vi "XNET.Cluster.Convert.Initialize.vi"(8 "error in":errorcluster, 10 "CAN Cluster":T1={"64bit Baud Rate"=125000, "Comment"="", "Name"="", "Transmit I/O Mode"=0, "64bit FD Baud Rate"=0} {"Transmit I/O Mode" items=["CAN 2.0", "CAN FD", "CAN FD+BRS"]}, 11 "database in":refnum<k21>) -> (0 "error out":errorcluster, 3 "cluster out":refnum<k21>)   [LabVIEW 2024, in "Diagnostics Addon Engine.lvlib"]
uses:
  Diagnostics Addon Engine.lvlib
  Types/XNET.Cluster.ctl
  <vilib>/xnet/xnet.llb/XNET Database Create (Cluster).vi
  <resource>/objmgr/xnet.rc
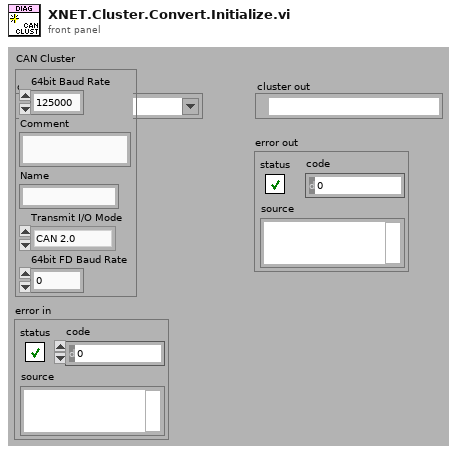
[diagram p1: front panel]
types:
  T1 = typedef "Diagnostics Addon Engine.lvlib/XNET.Cluster.ctl" = cluster{"64bit Baud Rate":u64, "Comment":string, "Name":string, "Transmit I/O Mode":u32, "64bit FD Baud Rate":u64}
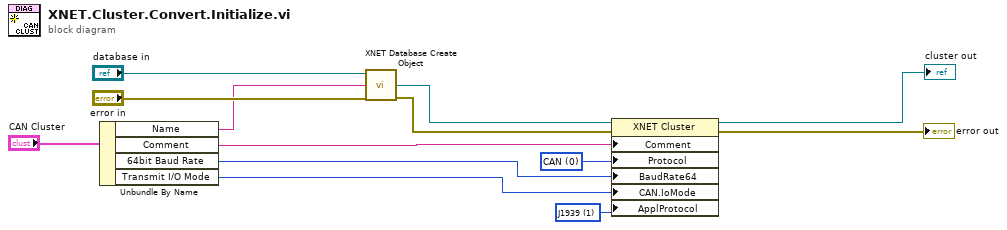
[diagram p0: block diagram]
diagram:
  w1 = u32 1 items=["None", "J1939"] ("Application Protocol")
  w2 = u32 0 items=["CAN", "FlexRay"] ("Protocol")
  n1 = Unbundle By Name("CAN Cluster") -> ("Name"=w10:string, "Comment"=w11:string, "64bit Baud Rate"=w4:u64, "Transmit I/O Mode"=w3:u32)
  n2 = call-poly <vilib>:"XNET Database Create Object.vi"("database in"="database in", "cluster name"=w10, "error in (no error)"="error in") -> ("cluster out"=w5:refnum<k21>, "error out"=w9:errorcluster)  [unwired: 10 in, 1 out]
  n3 = property class="XNET Cluster"(reference=w5, error in=w9, "Comment"=w11, "Protocol"=w2, "BaudRate64"=w4, "CAN.IoMode"=w3, "ApplProtocol"=w1) -> (reference out=→"cluster out":refnum<k21>, error out=→"error out":errorcluster)
